vi "Cursor Query.vi"(0 "RedPitaya connection in":refnum<k5>, 1 "Query":u16(ring) items=["Voltage at cursor", "time at cursor", "time between cursors", "voltage difference at 2 cursors", "freq between 2 cursors"], 2 "Cursor 1":u16, 3 "Cursor 2":u16, 5 "error in":errorcluster, 8 "Channel #":u16(ring)=1 items=["Channel 1"=1, "Channel 2"=2], 12 "timeout ms (2000)":i32=2000) -> (14 "RedPitaya connection out":refnum<k5>, 16 "Output string":string, 19 "error out":errorcluster)   [LabVIEW 2021, in "RedPitaya.lvlib"]
doc: "Returns specific information depending on cursor position from Red Pitaya. \n\nParameters you have to provide depending on query:\n-Voltage at cursor: channel #, cursor 1\n-Time at cursor: channel #\n-Time between cursors: cursor 1, cursor 2\n-Voltage difference at 2 cursors: channel #, cursor 1, cursor 2\n-Frequency between 2 cursors: cursor 1, cursor 2"
uses:
  RedPitaya.lvlib
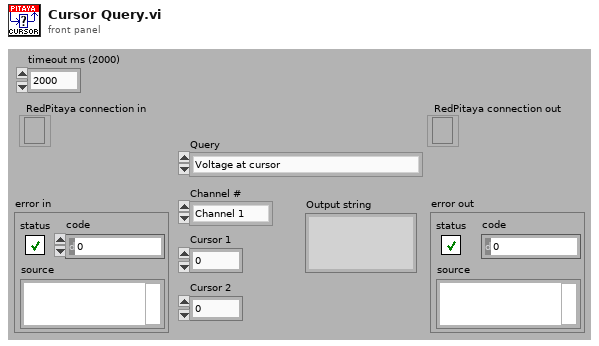
[diagram p1: front panel]
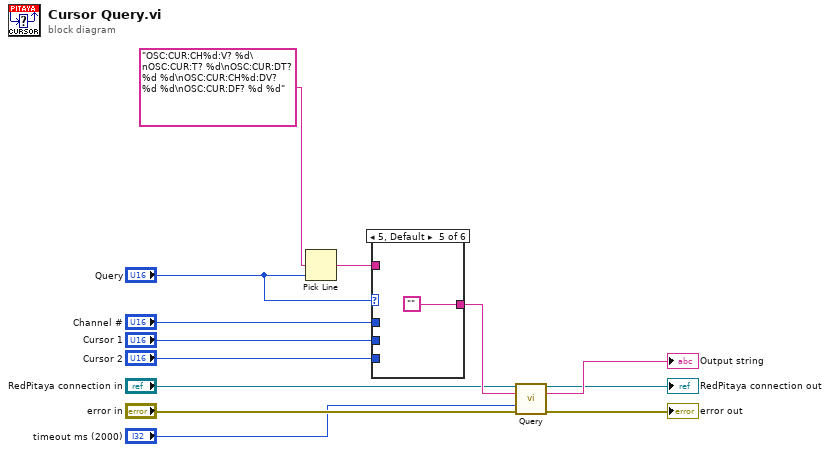
[diagram p0: block diagram]
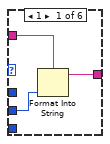
[diagram p2: hidden frame]
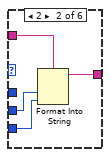
[diagram p3: hidden frame]
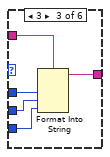
[diagram p4: hidden frame]
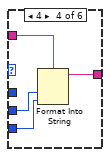
[diagram p5: hidden frame]
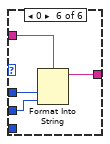
[diagram p6: hidden frame]
diagram:
  n1 = Pick Line(multi-line string="OSC:CUR:CH%d:V? %d\nOSC:CUR:T? %d\nOSC:CUR:DT? %d %d\nOSC:CUR:CH%d:DV? %d %d\nOSC:CUR:DF? %d %d", line index="Query") -> (output string=w10:string)  [unwired: 1 in]
  n2 = case shown="5, Default" "Query" {
    tunnel: [w16 w20 w25 w29 "" w34] -> w11
    tunnel: "Cursor 1" -> [w15 w18 w22 w28 _ w31]
    tunnel: w10 -> [w14 w19 w24 w27 _ w33]
    tunnel: "Cursor 2" -> [_ w17 w21 w26 _ _]
    tunnel: "Channel #" -> [_ _ w23 _ _ w32]
    frame 1 {
      n3 = Format Into String(format string=w14, w15) -> (resulting string=w16:string)  [unwired: 2 in, 1 out]
    }
    frame 2 {
      n4 = Format Into String(format string=w19, w18, w17) -> (resulting string=w20:string)  [unwired: 2 in, 1 out]
    }
    frame 3 {
      n5 = Format Into String(format string=w24, w23, w22, w21) -> (resulting string=w25:string)  [unwired: 2 in, 1 out]
    }
    frame 4 {
      n6 = Format Into String(format string=w27, w28, w26) -> (resulting string=w29:string)  [unwired: 2 in, 1 out]
    }
    frame 5, Default {
    }
    frame 0 {
      n7 = Format Into String(format string=w33, w32, w31) -> (resulting string=w34:string)  [unwired: 2 in, 1 out]
    }
  }
  n8 = call "Query.vi"("RedPitaya connection in"="RedPitaya connection in", "SCPI Query"=w11, "timeout ms (2000)"="timeout ms (2000)", "error in"="error in") -> ("RedPitaya connection out"=→"RedPitaya connection out":refnum<k5>, "data out"=→"Output string":string, "error out"=→"error out":errorcluster)  [unwired: 9 in]
